vi "ZStage_Move.vi"(0 "Position":sgl, 1 "Z_Wait":bool=TRUE) -> ()   [LabVIEW 2016]
uses:
  Utility/Global Constants.vi
  Utility/Global_Stage.vi
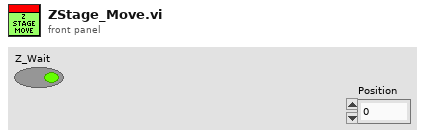
[diagram p1: front panel]
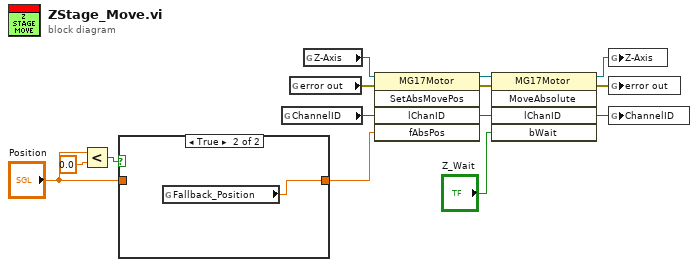
[diagram p0: block diagram]
diagram:
  n1 = Less?(x="Position", y=sgl 0.0) -> (x < y?=w3:bool)
  n2 = case shown="True" w3 {
    tunnel: [w15 w16] -> w2
    tunnel: "Position" -> [w15 _]
    frame False {
    }
    frame True {
      n3 = global read "Global Constants.vi" "Fallback_Position"() -> (w16:sgl)
    }
  }
  n4 = global read "Global_Stage.vi" "ChannelID"() -> (w8:i32)
  n5 = global read "Global Constants.vi" "error out"() -> (w7:errorcluster)
  n6 = global read "Global_Stage.vi" "Z-Axis"() -> (w10:refnum<k7>)
  n7 = invoke class="MG17Motor" method="SetAbsMovePos"(reference=w10, error in=w7, "lChanID"=w8, "fAbsPos"=w2) -> (reference out=w12:refnum<k7>, error out=w13:errorcluster, "lChanID"=w14:i32)  [unwired: 1 in, 2 out]
  n8 = invoke class="MG17Motor" method="MoveAbsolute"(reference=w12, error in=w13, "lChanID"=w14, "bWait"="Z_Wait") -> (reference out=w9:refnum<k7>, error out=w6:errorcluster, "lChanID"=w5:i32)  [unwired: 1 in, 2 out]
  n9 = global write "Global_Stage.vi" "Z-Axis"(w9) -> ()
  n10 = global write "Global Constants.vi" "error out"(w6) -> ()
  n11 = global write "Global_Stage.vi" "ChannelID"(w5) -> ()
